vi "Flush Data to Log File.vi"(8 "error in (no error)":errorcluster, 10 "Data Queue":refnum<queue>, 11 "Logging Configuration":T1) -> (0 "error out":errorcluster)   [LabVIEW 2013, in "Logging.lvlib"]
doc: "Flush the data queue of any pending data and write it to the log file. Close the TDMS file reference."
uses:
  Logging.lvlib
  Logging Configuration.ctl
  <vilib>/Waveform/WDTOps.llb/WDT Index Channel DBL.vi
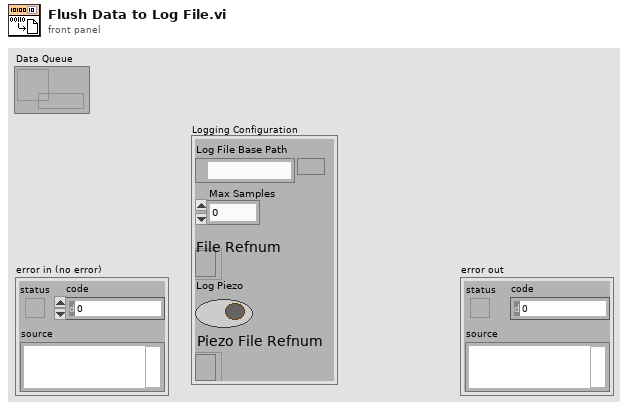
[diagram p1: front panel]
types:
  T1 = typedef "Logging.lvlib/Logging Configuration.ctl" = cluster{"Log File Base Path":path, "Max Samples":u32, "File Refnum":refnum<file>, "Log Piezo":bool, "Piezo File Refnum":refnum<file>}
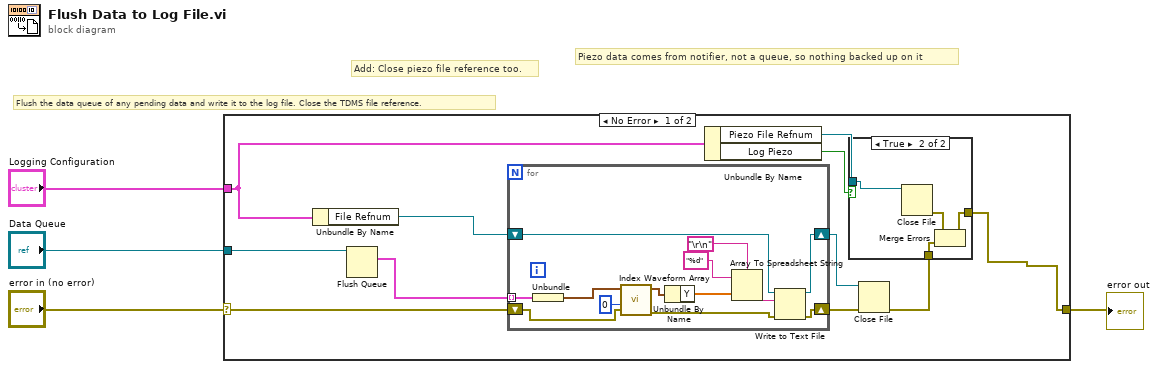
[diagram p0: block diagram]
diagram:
  # "Piezo data comes from notifier, not a queue, so nothing backed up on it"
  # "Add: Close piezo file reference too."
  # "Flush the data queue of any pending data and write it to the log file. Close the TDMS file reference."
  n1 = case shown="No Error" "error in (no error)" {
    selector: "error in (no error)" -> [w12 w34]
    tunnel: "Data Queue" -> [w13 _]
    tunnel: "Logging Configuration" -> [w9 _]
    tunnel: [w5 w34] -> w2
    frame No Error {
      n2 = Unbundle By Name(w9) -> ("File Refnum"=w14:refnum<file>)
      n3 = Flush Queue(queue=w13) -> (remaining elements=w15:cluster{"Array":waveform(dbl)[]}[])  [unwired: 1 in, 2 out]
      n4 = for {
        shift-right: [w23] -> w10
        shift-left: w14 -> [w24]
        shift-right: [w22] -> w11
        shift-left: w12 -> [w30]
        tunnel: w15 -> [w33] mode=indexing
        n5 = Unbundle(w33) -> ("Array"=w29:waveform(dbl)[])
        n6 = call-poly <vilib>:"Index Waveform Array.vi"("error in (no error)"=w30, "index"=0, "waveform array"=w29) -> ("error out"=w26:errorcluster, "waveform"=w31:waveform(dbl))  [unwired: 7 in]
        n7 = Unbundle By Name(w31) -> ("Y"=w25:dbl[])
        n8 = Array To Spreadsheet String(delimiter (Tab)="\r\n", array=w25, 3:"%d" ("format string")) -> (spreadsheet string=w28:string)
        n9 = Write to Text File(file (use dialog)=w24, text=w28, error in=w26) -> (refnum out=w23:refnum<file>, error out=w22:errorcluster)  [unwired: 1 in, 1 out]
      }
      n10 = Unbundle By Name(w9) -> ("Piezo File Refnum"=w7:refnum<file>, "Log Piezo"=w8:bool)
      n11 = Close File(refnum=w10, error in=w11) -> (error out=w6:errorcluster)  [unwired: 1 out]
      n12 = case shown="True" w8 {
        tunnel: w7 -> [_ w20]
        tunnel: [w16 w17] -> w5
        tunnel: w6 -> [w16 w18]
        frame False {
        }
        frame True {
          n13 = Close File(refnum=w20) -> (error out=w19:errorcluster)  [unwired: 1 in, 1 out]
          n14 = Merge Errors(w19, w18) -> (w17:errorcluster)
        }
      }
    }
    frame Error {
    }
  }
  "error out" <- w2
